vi "REF Single  Name to ref convert.vi"(11 "name":string) -> (3 "First REF":refnum<vi>)   [LabVIEW 2020]
uses:
  PCT FGV CMD.ctl
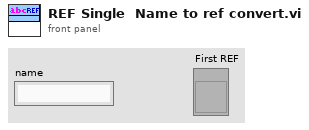
[diagram p1: front panel]
types:
  T1 = typedef "PCT FGV CMD.ctl" = enum16{"INIT", "GET", "SET"}
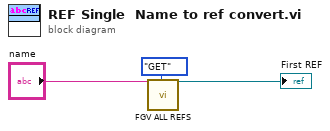
[diagram p0: block diagram]
diagram:
  n1 = call "FGV ALL REFS.vi"("name"="name", "CMD"=PCT_FGV_CMD."GET") -> ("Ctl Refnum out"=→"First REF":refnum<vi>)  [unwired: 25 in]
